vi "Launch Nested Actors.vi"(8 "error in (no error)":errorcluster, 11 "AMS Gas in":refnum<class "AMS Gas.lvclass">) -> (0 "error out":errorcluster, 3 "AMS Gas out":refnum<class "AMS Gas.lvclass">)   [LabVIEW 2015, in "AMS UI.lvlib" / "AMS Gas.lvclass"]
uses:
  AMS Gas.lvclass
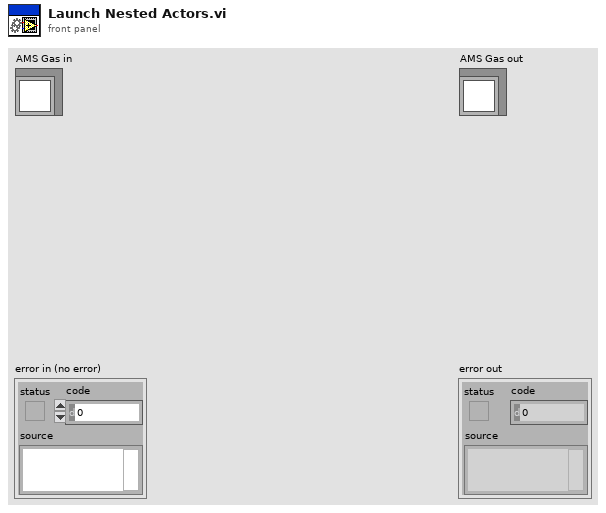
[diagram p1: front panel]
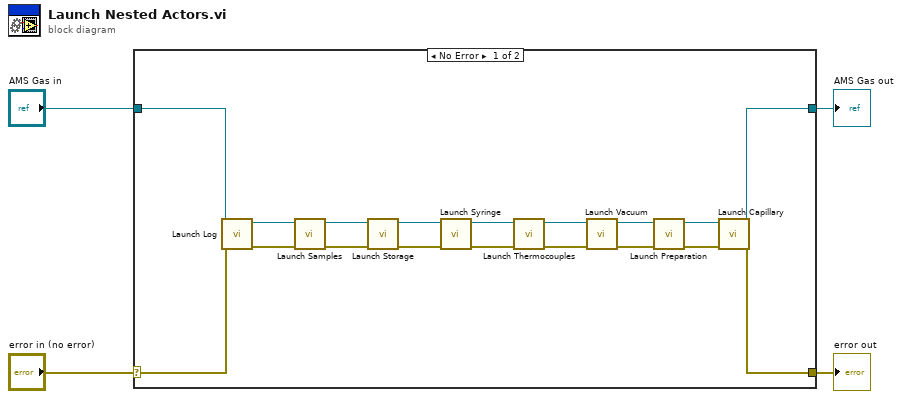
[diagram p0: block diagram]
diagram:
  n1 = case shown="No Error" "error in (no error)" {
    selector: "error in (no error)" -> [w11 w24]
    tunnel: [w8 w24] -> w3
    tunnel: [w9 w23] -> w1
    tunnel: "AMS Gas in" -> [w12 w23]
    frame No Error {
      n2 = call "Launch Log.vi"("error in (no error)"=w11, "AMS Gas in"=w12) -> ("error out"=w17:errorcluster, "AMS Gas out"=w22:refnum<class "AMS Gas.lvclass">)  [unwired: 8 in]
      n3 = call "Launch Samples.vi"("error in (no error)"=w17, "AMS Gas in"=w22) -> ("error out"=w16:errorcluster, "AMS Gas out"=w21:refnum<class "AMS Gas.lvclass">)  [unwired: 8 in]
      n4 = call "Launch Storage.vi"("error in (no error)"=w16, "AMS Gas in"=w21) -> ("error out"=w15:errorcluster, "AMS Gas out"=w20:refnum<class "AMS Gas.lvclass">)  [unwired: 8 in]
      n5 = call "Launch Syringe.vi"("error in (no error)"=w15, "AMS Gas in"=w20) -> ("error out"=w14:errorcluster, "AMS Gas out"=w19:refnum<class "AMS Gas.lvclass">)  [unwired: 8 in]
      n6 = call "Launch Thermocouples.vi"("error in (no error)"=w14, "AMS Gas in"=w19) -> ("error out"=w13:errorcluster, "AMS Gas out"=w18:refnum<class "AMS Gas.lvclass">)  [unwired: 8 in]
      n7 = call "Launch Vacuum.vi"("error in (no error)"=w13, "AMS Gas in"=w18) -> ("error out"=w6:errorcluster, "AMS Gas out"=w10:refnum<class "AMS Gas.lvclass">)  [unwired: 8 in]
      n8 = call "Launch Preparation.vi"("error in (no error)"=w6, "AMS Gas in"=w10) -> ("error out"=w5:errorcluster, "AMS Gas out"=w7:refnum<class "AMS Gas.lvclass">)  [unwired: 8 in]
      n9 = call "Launch Capillary.vi"("error in (no error)"=w5, "AMS Gas in"=w7) -> ("error out"=w8:errorcluster, "AMS Gas out"=w9:refnum<class "AMS Gas.lvclass">)  [unwired: 8 in]
    }
    frame Error {
    }
  }
  "error out" <- w3
  "AMS Gas out" <- w1
